vi "EXAMPLE_1.vi"() -> ()   [LabVIEW 2013]
uses:
  <vilib>/Utility/error.llb/DialogType.ctl
  <vilib>/Analysis/baseanly.llb/Mean (DBL).vi
  <instrlib>/ZBOX_IS/ZBOX_IS.lvlib
  <vilib>/Analysis/NI_AALBase.lvlib
panel:
  out "Battery Status":dbl
  out "Battery Voltage":dbl
  in  "DATA STREAMING":bool=TRUE
  in  "supply":bool
  in  "ChB":u8(slide) scale=0.0..3.0
  in  "ChA":u8(slide) scale=0.0..3.0
  out "Status":string
  out "Front End":string
  out "Connected":bool
  out "Magnitude,   ohm":cluster{"freqs":dbl[], dbl[]}(graph)
  out "Phase, deg":cluster{"freqs":dbl[], dbl[]}(graph)
  out "level":T1={"Slide 5"={844, 3164}, "max OL 10"=FALSE, "max OL 9"=FALSE, "Slide 4"={867, 3199}, "max OL 8"=FALSE, "max OL 7"=FALSE} {"Slide 4" scale=0.0..4096.0; "Slide 5" scale=0.0..4096.0}
  in  "stop":bool
  out "DLL version":string
  out "Device":string
  in  "signal":u32(slide)=50 scale=0.0..100.0
  # "10"
  # "5"
  # "2"
  # "1"
  # "10"
  # "5"
  # "2"
  # "1"
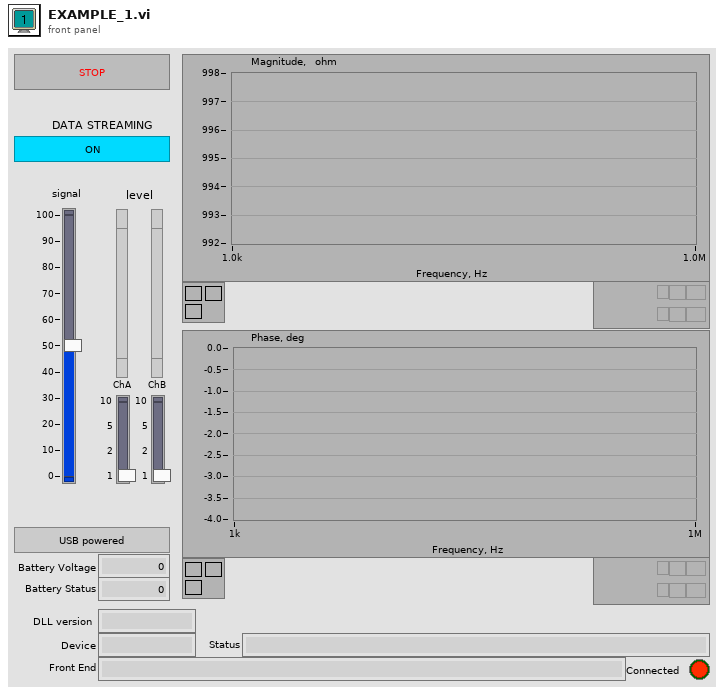
[diagram p1: front panel]
types:
  T1 = cluster{"Slide 5":cluster{u16, u16}, "max OL 10":bool, "max OL 9":bool, "Slide 4":cluster{u16, u16}, "max OL 8":bool, "max OL 7":bool}
  T2 = typedef "DialogType.ctl" = u16
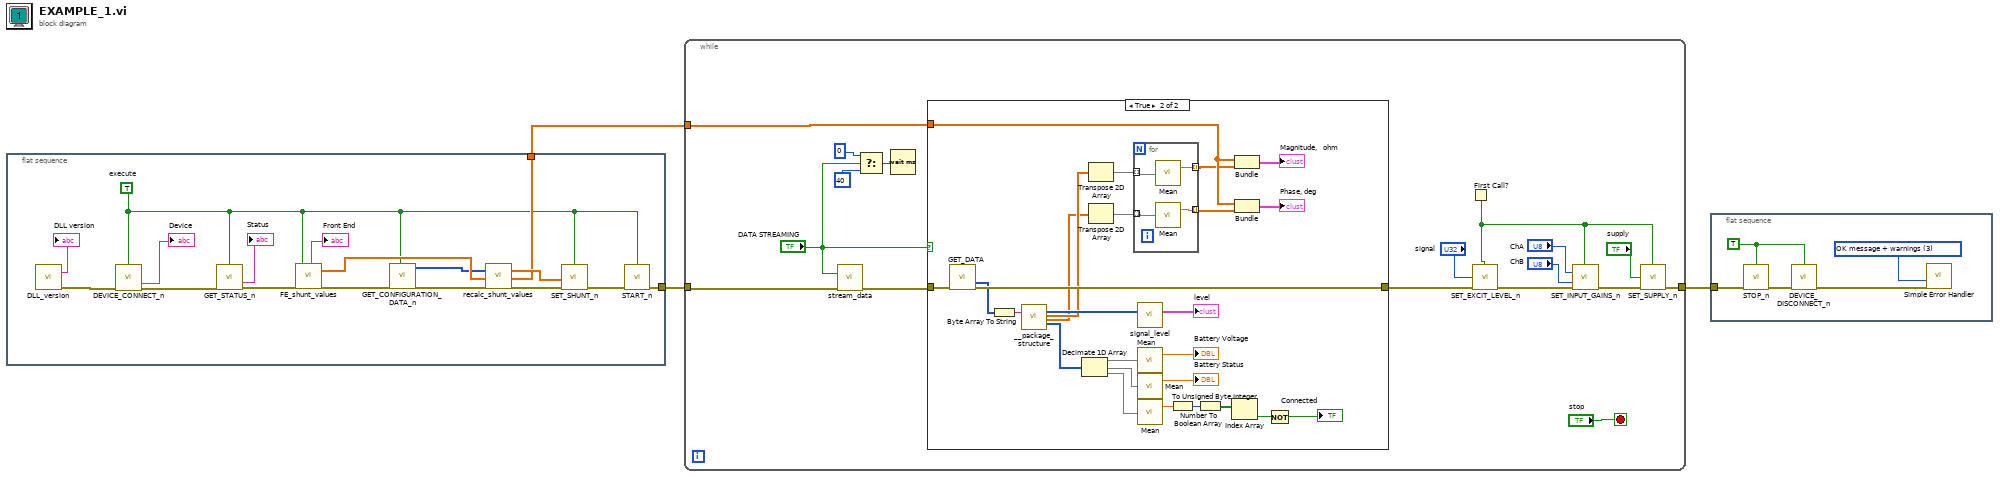
[diagram p0: block diagram]
diagram:
  n1 = flat-sequence {
    tunnel: [w16] -> w2
    tunnel: [w11] -> w1
    frame #0 {
      w6 = TRUE  # execute
      n2 = call <instrlib>:"DLL_version.vi"() -> ("DLL version"=→"DLL version":string, "error out"=w4:errorcluster)  [unwired: 13 in, 1 out]
      n3 = call <instrlib>:"DEVICE_CONNECT_n.vi"("execute"=w6, "error in (no error)"=w4) -> ("serial no"=→"Device":string, "error out"=w19:errorcluster)  [unwired: 10 in, 2 out]
      n4 = call <instrlib>:"GET_STATUS_n.vi"("execute"=w6, "error in (no error)"=w19) -> ("serial no"=→"Status":string, "error out"=w15:errorcluster)  [unwired: 10 in, 2 out]
      n5 = call <instrlib>:"FE_shunt_values.vi"("error in (no error)"=w15, "execute"=w6) -> ("shunt"=→"Front End":string, "FE_shunt_data"=w14:sgl[], "error out"=w10:errorcluster)  [unwired: 14 in, 1 out]
      n6 = call <instrlib>:"GET_CONFIGURATION_DATA_n.vi"("error in (no error)"=w10, "execute"=w6) -> ("DFTBins"=w8:u16[], "error out"=w9:errorcluster)  [unwired: 7 in, 9 out]
      n7 = call <instrlib>:"recalc_shunt_values.vi"("DFTBins"=w8, "FE_shunt_data"=w14, "error in (no error)"=w9) -> ("shunt"=w12:cdb[], "freqs"=w11:dbl[], "error out"=w13:errorcluster)  [unwired: 13 in, 1 out]
      n8 = call <instrlib>:"SET_SHUNT_n.vi"("execute"=w6, "SHUNT values"=w12, "error in (no error)"=w13) -> ("error out"=w7:errorcluster)  [unwired: 11 in, 1 out]
      n9 = call <instrlib>:"START_n.vi"("execute"=w6, "error in (no error)"=w7) -> ("error out"=w16:errorcluster)  [unwired: 12 in, 1 out]
    }
  }
  n10 = while {
    tunnel: w2 -> [w26]
    tunnel: [w28] -> w3
    tunnel: w1 -> [w29]
    stop <- "stop" stop-if-true
    n11 = call <instrlib>:"stream_data.vi"("DATA STREAMING"="DATA STREAMING", "error in (no error)"=w26) -> ("error out"=w25:errorcluster)  [unwired: 13 in]
    n12 = Select(t=u32 0, s="DATA STREAMING", f=u32 40 ("wait")) -> (s? t:f=w23:u32)
    n13 = Wait (ms)(milliseconds to wait=w23) -> ()  [unwired: 1 out]
    n14 = case shown="True" "DATA STREAMING" {
      tunnel: w29 -> [_ w64]
      tunnel: w25 -> [w38 w63]
      tunnel: [w38 w62] -> w30
      frame False {
      }
      frame True {
        n15 = call <instrlib>:"GET_DATA.vi"("error in (no error)"=w63) -> ("BytePtr"=w60:u8[], "error out"=w62:errorcluster)  [unwired: 12 in, 1 out]
        n16 = Byte Array To String(unsigned byte array=w60) -> (string=w61:string)
        n17 = call <instrlib>:"__package_structure.vi"("data"=w61) -> ("max_min"=w58:u16[], "M"=w53:sgl[][], "Ph"=w52:sgl[][], "status"=w46:u16[])  [unwired: 8 in, 7 out]
        n18 = Decimate 1D Array(w46) -> (w43:u16[], w44:u16[], w45:u16[])
        n19 = Transpose 2D Array(2D array=w53) -> (transposed array=w56:sgl[][])
        n20 = Transpose 2D Array(2D array=w52) -> (transposed array=w57:sgl[][])
        n21 = for {
          tunnel: w56 -> [w68] mode=indexing
          tunnel: [w67] -> w55 mode=indexing
          tunnel: w57 -> [w65] mode=indexing
          tunnel: [w66] -> w54 mode=indexing
          n22 = call-poly <vilib>:"Mean.vi"("X"=w68) -> ("mean"=w67:dbl)  [unwired: 1 out]
          n23 = call-poly <vilib>:"Mean.vi"("X"=w65) -> ("mean"=w66:dbl)  [unwired: 1 out]
        }
        n24 = call <instrlib>:"signal_level.vi"("data U16"=w58) -> ("level"=→"level":T1)  [unwired: 14 in]
        n25 = call-poly <vilib>:"Mean.vi"("X"=w43) -> ("mean"=→"Battery Voltage":dbl)  [unwired: 1 out]
        n26 = call-poly <vilib>:"Mean.vi"("X"=w44) -> ("mean"=→"Battery Status":dbl)  [unwired: 1 out]
        n27 = call-poly <vilib>:"Mean.vi"("X"=w45) -> ("mean"=w49:dbl)  [unwired: 1 out]
        n28 = To Unsigned Byte Integer(number=w49) -> (unsigned 8bit integer=w48:u8)
        n29 = Number To Boolean Array(number=w48) -> (Boolean array=w47:bool[])
        n30 = Index Array(array=w47) -> (element=w40:bool)  [unwired: 1 in]
        n31 = Bundle("freqs"=w64, w55) -> (→"Magnitude,   ohm":cluster{"freqs":dbl[], dbl[]})  [unwired: 1 in]
        n32 = Bundle("freqs"=w64, w54) -> (→"Phase, deg":cluster{"freqs":dbl[], dbl[]})  [unwired: 1 in]
        n33 = Not(x=w40) -> (.not. x?=→"Connected":bool)
      }
    }
    n34 = First Call?() -> (First Call?: T/F=w27:bool)
    n35 = call <instrlib>:"SET_EXCIT_LEVEL_n.vi"("execute"=w27, "Level"="signal", "error in (no error)"=w30) -> ("error out"=w35:errorcluster)  [unwired: 11 in, 1 out]
    n36 = call <instrlib>:"SET_INPUT_GAINS_n.vi"("execute"=w27, "G1"="ChA", "G2"="ChB", "error in (no error)"=w35) -> ("error out"=w32:errorcluster)  [unwired: 10 in, 1 out]
    n37 = call <instrlib>:"SET_SUPPLY_n.vi"("execute"=w27, "supply"="supply", "error in (no error)"=w32) -> ("error out"=w28:errorcluster)  [unwired: 11 in, 1 out]
  }
  n38 = flat-sequence {
    tunnel: w3 -> [w73]
    frame #0 {
      w69 = T2 3 items=["no dialog", "OK message", "continue or stop message", "OK message + warnings", "continue/stop + warnings"] ("type of dialog (OK msg:1)")
      w71 = TRUE ("execute")
      n39 = call <instrlib>:"STOP_n.vi"("execute"=w71, "error in (no error)"=w73) -> ("error out"=w72:errorcluster)  [unwired: 12 in, 1 out]
      n40 = call <instrlib>:"DEVICE_DISCONNECT_n.vi"("execute"=w71, "error in (no error)"=w72) -> ("error out"=w70:errorcluster)  [unwired: 12 in, 1 out]
      n41 = call <vilib>:"Simple Error Handler.vi"("type of dialog (OK msg:1)"=w69, "error in (no error)"=w70) -> ()  [unwired: 3 in, 5 out]
    }
  }
